vi "Calculate Makespan.vi"(10 "Gannt Chart Out":T1[][](array[typedef]), 11 "Number of Jobs":i32) -> (3 "Makespan":i32)   [LabVIEW 2013, in "GA.lvclass"]
uses:
  GA.lvclass
  Controls/GanntChart_Element.ctl
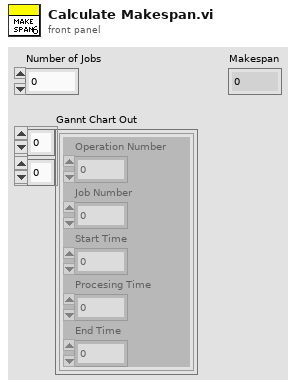
[diagram p1: front panel]
types:
  T1 = typedef "GanntChart_Element.ctl" = cluster{"Operation Number":i32, "Job Number":i32, "Start Time":i32, "Procesing Time":u16, "End Time":i32}
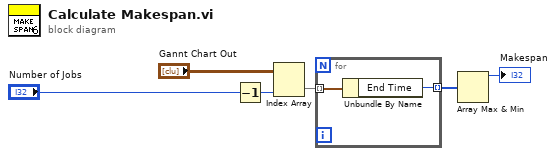
[diagram p0: block diagram]
diagram:
  n1 = Decrement(x="Number of Jobs") -> (x-1=w1:i32)
  n2 = Index Array(array="Gannt Chart Out", index (col)=w1) -> (element=w3:T1[])  [unwired: 1 in]
  n3 = for {
    tunnel: w3 -> [w8] mode=indexing
    tunnel: [w7] -> w2 mode=indexing
    n4 = Unbundle By Name(w8) -> ("End Time"=w7:i32)
  }
  n5 = Array Max & Min(array=w2) -> (max value=→"Makespan":i32)  [unwired: 3 out]
